vi "peg_leg_map_button_to_state.vi"(10 "Button":bool, 11 "peg_leg_state":T1=enum."down") -> ()   [LabVIEW 2011]
uses:
  peg_leg_state.ctl
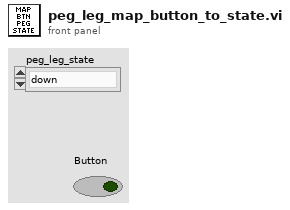
[diagram p1: front panel]
types:
  T1 = typedef "peg_leg_state.ctl" = enum16{"up", "down", "unfold", "manual"}
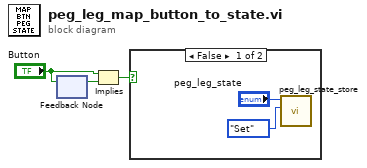
[diagram p0: block diagram]
diagram:
  n1 = feedback-in #1("Button") -> ()
  n2 = feedback #1() -> (w2:bool)  [unwired: 1 in]
  n3 = Implies(1:w2, 2:"Button") -> (0:w1:bool)
  n4 = case shown="False" w1 {
    frame False {
      n5 = call "peg_leg_state_store.vi"("data_store_mode"=enum16{"Set", "Get"}."Set", "peg_leg_state"="peg_leg_state") -> ()  [unwired: 8 in, 2 out]
    }
    frame True {
    }
  }
